vi "timer.vi"(10 "Target Time (ms)":u32, 11 "Mode":enum16{"Set", "Read"}(ring)) -> (3 "Passed":bool)   [LabVIEW 2017]
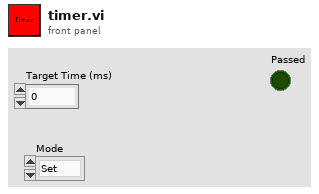
[diagram p1: front panel]
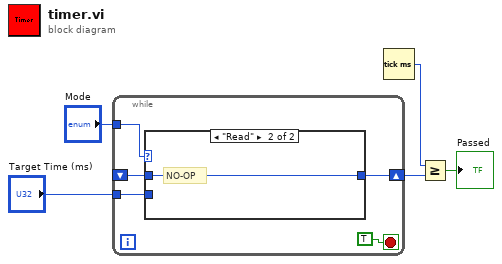
[diagram p0: block diagram]
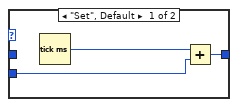
[diagram p2: hidden frame]
diagram:
  n1 = while {
    tunnel: "Mode" -> [w9]
    tunnel: "Target Time (ms)" -> [w8]
    shift-right: [w7] -> w2
    shift-left: _ -> [w6]
    stop <- TRUE stop-if-true
    n2 = case shown="\"Read\"" w9 {
      tunnel: w8 -> [w12 _]
      tunnel: [w11 w14] -> w7
      tunnel: w6 -> [_ w14]
      frame "Set", Default {
        n3 = Tick Count (ms)() -> (millisecond timer value=w13:u32)
        n4 = Add(x=w13, y=w12) -> (x+y=w11:u32)
      }
      frame "Read" {
        # "NO-OP"
      }
    }
  }
  n5 = Tick Count (ms)() -> (millisecond timer value=w3:u32)
  n6 = Greater Or Equal?(x=w3, y=w2) -> (x >= y?=→"Passed":bool)
